vi "SubVI_Func_Calibragem.vi"(1 "Tensão SAT Fotodetector (V)":dbl, 2 "Freq_atual":dbl, 3 "Canal":i32(ring) items=["1", "2"], 4 "Osciloscópio":refnum<visa-resource-name>="GPIB0::1::INSTR") -> (0 "Osciloscópio out":refnum<visa-resource-name>)   [LabVIEW 2018]
uses:
  349eac8f-d71b-46e2-b8b6-b89c51f9ffec.vi
  88633d66-928a-4884-bfe4-ed0cc3c1c186.vi
  d5c54376-684d-44cb-b049-75f578ed463c.vi
  164e57bc-af4c-43c9-a344-bbe8c37d70be.vi
  beef57f8-5705-44eb-9d3c-e7656767c87b.vi
  445fce54-bd66-4484-b71a-0e2296e8cbee.vi
  11d1bd32-39af-459b-a544-a1d0d28f5ea3.vi
  ff351943-6c23-4d5c-97eb-6a29b78aebe1.vi
panel:
  out "VISA resource name out 2":refnum<visa-resource-name>
  out "VISA resource name out":refnum<visa-resource-name>
  out "AVG":dbl
  out "Escala":string
  out "VMIN":dbl
  out "VMAX":dbl
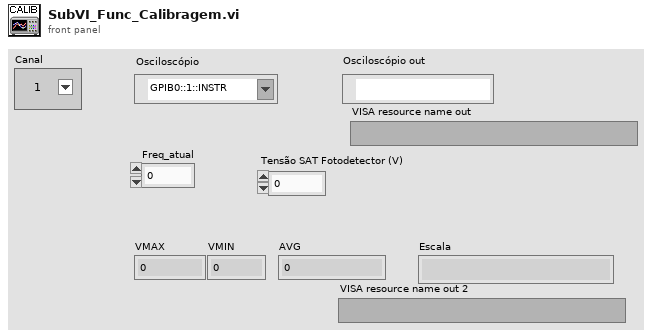
[diagram p1: front panel]
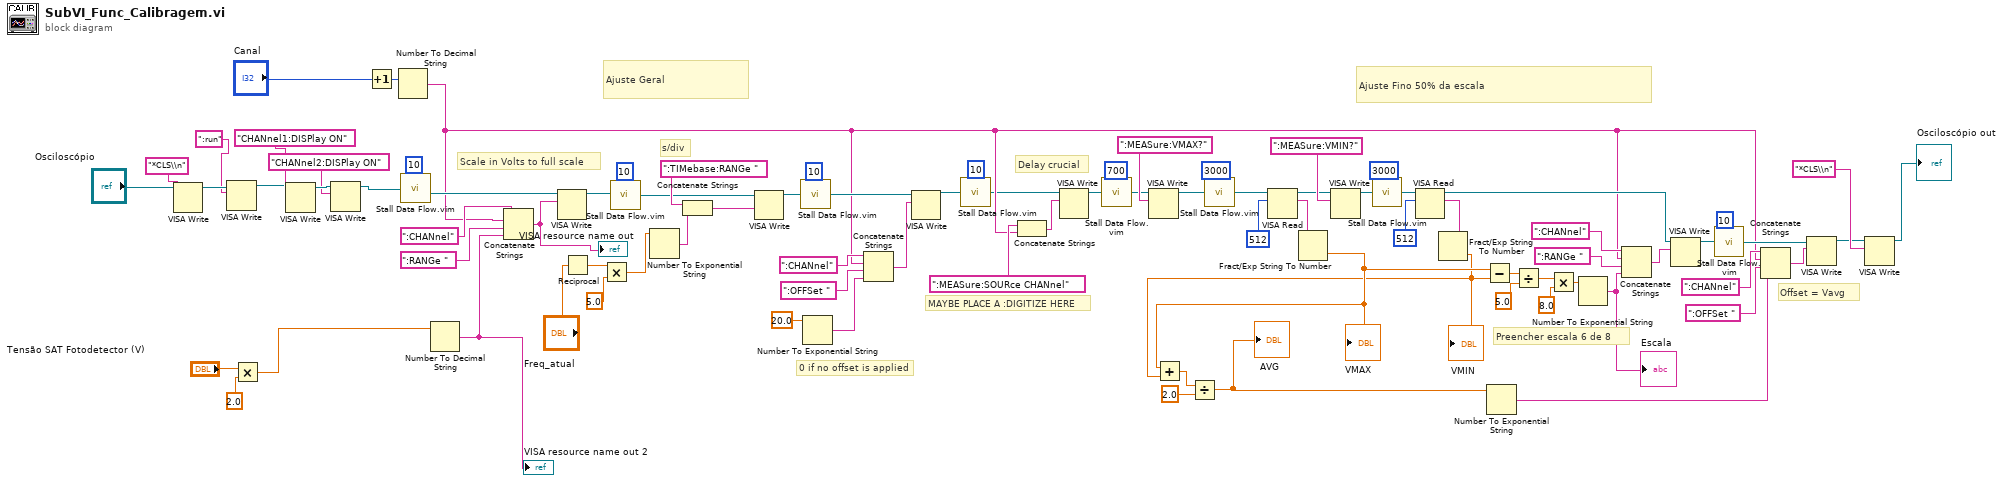
[diagram p0: block diagram]
diagram:
  # "MAYBE PLACE A :DIGITIZE HERE"
  # "0 if no offset is applied"
  # "Delay crucial"
  # "Offset = Vavg"
  # "Preencher escala 6 de 8"
  # "s/div"
  # "Scale in Volts to full scale"
  # "Ajuste Fino 50% da escala"
  # "Ajuste Geral"
  n1 = VISA Write(VISA resource name="Osciloscópio", write buffer="*CLS\\n") -> (VISA resource name out=w3:refnum<visa-resource-name>)  [unwired: 1 in, 2 out]
  n2 = VISA Write(VISA resource name=w3, write buffer=":run") -> (VISA resource name out=w2:refnum<visa-resource-name>)  [unwired: 1 in, 2 out]
  n3 = Multiply(x="Tensão SAT Fotodetector (V)", y=2.0) -> (x*y=w15:dbl)
  n4 = VISA Write(VISA resource name=w2, write buffer="CHANnel1:DISPlay ON") -> (VISA resource name out=w6:refnum<visa-resource-name>)  [unwired: 1 in, 2 out]
  n5 = VISA Write(VISA resource name=w6, write buffer="CHANnel2:DISPlay ON") -> (VISA resource name out=w5:refnum<visa-resource-name>)  [unwired: 1 in, 2 out]
  n6 = Increment(x="Canal") -> (x+1=w61:i32)
  n7 = Number To Decimal String(number=w61) -> (decimal integer string=w28:string)  [unwired: 1 in]
  n8 = call "Stall Data Flow.vim"("value in"=w5, "milliseconds to wait"=u32 10) -> ("value out"=w46:refnum<visa-resource-name>)  [unwired: 1 out]
  n9 = Number To Decimal String(number=w15) -> (decimal integer string=w14:string)  [unwired: 1 in]
  "VISA resource name out 2" <- w14
  n10 = Concatenate Strings(":CHANnel" ("write buffer"), w28, ":RANGe " ("write buffer"), w14) -> (w16:string)
  "VISA resource name out" <- w16
  n11 = VISA Write(VISA resource name=w46, write buffer=w16) -> (VISA resource name out=w17:refnum<visa-resource-name>)  [unwired: 1 in, 2 out]
  n12 = Reciprocal(x="Freq_atual") -> (1/x=w67:dbl)
  n13 = Multiply(x=w67, y=5.0) -> (x*y=w68:dbl)
  n14 = call "Stall Data Flow.vim"("value in"=w17, "milliseconds to wait"=u32 10) -> ("value out"=w38:refnum<visa-resource-name>)  [unwired: 1 out]
  n15 = Number To Exponential String(number=w68) -> (E-format string=w83:string)  [unwired: 3 in]
  n16 = Concatenate Strings(":TIMebase:RANGe " ("write buffer"), w83) -> (w84:string)
  n17 = VISA Write(VISA resource name=w38, write buffer=w84) -> (VISA resource name out=w35:refnum<visa-resource-name>)  [unwired: 1 in, 2 out]
  n18 = call "Stall Data Flow.vim"("value in"=w35, "milliseconds to wait"=u32 10) -> ("value out"=w34:refnum<visa-resource-name>)  [unwired: 1 out]
  n19 = Number To Exponential String(number=20.0) -> (E-format string=w48:string)  [unwired: 3 in]
  n20 = Concatenate Strings(":CHANnel" ("write buffer"), w28, ":OFFSet " ("write buffer"), w48) -> (w82:string)
  n21 = VISA Write(VISA resource name=w34, write buffer=w82) -> (VISA resource name out=w40:refnum<visa-resource-name>)  [unwired: 1 in, 2 out]
  n22 = call "Stall Data Flow.vim"("value in"=w40, "milliseconds to wait"=u32 10) -> ("value out"=w27:refnum<visa-resource-name>)  [unwired: 1 out]
  n23 = Concatenate Strings(":MEASure:SOURce CHANnel" ("write buffer"), w28) -> (w29:string)
  n24 = VISA Write(VISA resource name=w27, write buffer=w29) -> (VISA resource name out=w25:refnum<visa-resource-name>)  [unwired: 1 in, 2 out]
  n25 = call "Stall Data Flow.vim"("value in"=w25, "milliseconds to wait"=u32 700) -> ("value out"=w24:refnum<visa-resource-name>)  [unwired: 1 out]
  n26 = VISA Write(VISA resource name=w24, write buffer=":MEASure:VMAX?") -> (VISA resource name out=w9:refnum<visa-resource-name>)  [unwired: 1 in, 2 out]
  n27 = call "Stall Data Flow.vim"("value in"=w9, "milliseconds to wait"=u32 3000) -> ("value out"=w8:refnum<visa-resource-name>)  [unwired: 1 out]
  n28 = VISA Read(VISA resource name=w8, byte count=u32 512) -> (VISA resource name out=w77:refnum<visa-resource-name>, read buffer=w75:string)  [unwired: 1 in, 2 out]
  n29 = Fract/Exp String To Number(string=w75) -> (number=w44:dbl)  [unwired: 3 in, 1 out]
  "VMAX" <- w44
  n30 = VISA Write(VISA resource name=w77, write buffer=":MEASure:VMIN?") -> (VISA resource name out=w13:refnum<visa-resource-name>)  [unwired: 1 in, 2 out]
  n31 = call "Stall Data Flow.vim"("value in"=w13, "milliseconds to wait"=u32 3000) -> ("value out"=w12:refnum<visa-resource-name>)  [unwired: 1 out]
  n32 = VISA Read(VISA resource name=w12, byte count=u32 512) -> (VISA resource name out=w71:refnum<visa-resource-name>, read buffer=w74:string)  [unwired: 1 in, 2 out]
  n33 = Fract/Exp String To Number(string=w74) -> (number=w43:dbl)  [unwired: 3 in, 1 out]
  "VMIN" <- w43
  n34 = Add(x=w44, y=w43) -> (x+y=w42:dbl)
  n35 = Divide(x=w42, y=2.0) -> (x/y=w21:dbl)
  "AVG" <- w21
  n36 = Subtract(x=w44, y=w43) -> (x-y=w73:dbl)
  n37 = Number To Exponential String(number=w21) -> (E-format string=w53:string)  [unwired: 3 in]
  n38 = Divide(x=w73, y=5.0) -> (x/y=w65:dbl)
  n39 = Multiply(x=w65, y=8.0) -> (x*y=w63:dbl)
  n40 = Number To Exponential String(number=w63) -> (E-format string=w56:string)  [unwired: 3 in]
  "Escala" <- w56
  n41 = Concatenate Strings(":CHANnel" ("write buffer"), w28, ":RANGe " ("write buffer"), w56) -> (w76:string)
  n42 = VISA Write(VISA resource name=w71, write buffer=w76) -> (VISA resource name out=w32:refnum<visa-resource-name>)  [unwired: 1 in, 2 out]
  n43 = call "Stall Data Flow.vim"("value in"=w32, "milliseconds to wait"=u32 10) -> ("value out"=w31:refnum<visa-resource-name>)  [unwired: 1 out]
  n44 = Concatenate Strings(":CHANnel" ("write buffer"), w28, ":OFFSet " ("write buffer"), w53) -> (w70:string)
  n45 = VISA Write(VISA resource name=w31, write buffer=w70) -> (VISA resource name out=w19:refnum<visa-resource-name>)  [unwired: 1 in, 2 out]
  n46 = VISA Write(VISA resource name=w19, write buffer="*CLS\\n") -> (VISA resource name out=→"Osciloscópio out":refnum<visa-resource-name>)  [unwired: 1 in, 2 out]
